vi "PacificPowerSource.vi"() -> ()   [LabVIEW 2018, in "Visualization.lvlib" / "VisualizeAcPwr.lvclass"]
doc: "This VI listens for any measurement data associated with the provided PluginName and displays it to the user for analysis. The display is only suitable for data coming from the RoomAlert Plugin."
uses:
  VisualizeAcPwr.lvclass
  ChromaPowerSupply/Loop Parameters.ctl
  VisualizeBase/VisualizeBase_class/SubVIs/VisualizationOptions.ctl
  <vilib>/Utility/miscctls.llb/LVRectTypeDef.ctl
  AcPwr/AcPwrPlugins/PacificPowerSourceClass/TypeDefs/Device(s)Settings.ctl
  AcPwr/AcPwrPlugins/PacificPowerSourceClass/TypeDefs/Measurements.ctl
  AcPwr/AcPwrPlugins/PacificPowerSourceClass/TypeDefs/MeasurementType.ctl
  AcPwr/AcPwrShared/clMeasurmentData.ctl
  AcPwr/AcPwrPlugins/AcPwrBaseClass/TypeDefs/SetParameterInputs.ctl
  <vilib>/event_ctls.llb/usereventprio.ctl
  VisualizeBase/VisualizeBase_class/Requests/VisUserEventType.ctl
  <vilib>/Utility/error.llb/Error Cluster From Error Code.vi
  <vilib>/ErrorRing/Error Ring.xnode
  <userlib>/NIST/NISTErrorLib/NISTErrorLib.lvlib
  VisualizeBase/VisualizeBase_class/VisualizeBase.lvclass
  TestClass/Test.lvclass
  Sensor/VisualizeSensor.lvclass
  StatusAndLog/VisualizeStatus.lvclass
  AcPwr/AcPwrShared/AcPwrShared.lvlib
  AcPwr/AcPwrModule/AcPwrModule.lvlib
  AcPwr/AcPwrPlugins/AcPwrPlugins.lvlib
  AcPwr/AcPwrPlugins/AcPwrBaseClass/AcPwrBase.lvclass
  AcPwr/AcPwrPlugins/PacificPowerSourceClass/PacificPowerSource.lvclass
panel:
  out "Chart#":i32
  out "MeasChannels":string[](array[string])
  out "Writetime":u32 caption="Sample Write Time(ms)"
  out "ExitHelperLoops?":bool
  in  "Display":enum16{"Raw Data", "Voltage Vs Current"}(ring)
  in  "btnPause":bool
  in  "INIFilePath":path
  in  "ModuleID":i32
  in  "Log Data":bool=TRUE
  in  "btnStop":bool
  in  "btnReset":bool
  in  "btnClearTest":bool
  in  "btnStopModule":bool
  out "XY Graph":cluster{dbl[], dbl[]}(graph)
  out "Chart":waveform(dbl)[](graph)=[{"t0"=timestamp(3657200531.6397257 s since 1904-01-01), "dt"=1.0, "Y"=[46.19]}, {"t0"=timestamp(3657200531.6397257 s since 1904-01-01), "dt"=1.0, "Y"=[2.0]}, {"t0"=timestamp(3657200531.6397257 s since 1904-01-01), "dt"=1.0, "Y"=[60.0]}]
  in  "Current":bool
  in  "Voltage":bool
  in  "Current (A)":dbl
  in  "Voltage (V)":dbl
  in  "btnStopParameterLoop":bool
  in  "btnRunParamLoop":bool
  in  "Loop Parameters":T1={"Parameter"=enum."Voltage", "Start Value"=5.0, "Increment"=1.0, "Interval (s)"=3.0, "# Iterations"=6, "End Value"=10.0} {"# Iterations" min=1; "Increment" format="%#.4f"}
  out "ErrorArray":errorcluster[](array[cluster])
  out "Incorrect DataType?":bool
  out "String Results":string
  in  "PluginName":string="Sensor.RoomAlert1"
  # "Set Parameter"
  # "Parameter Looping"
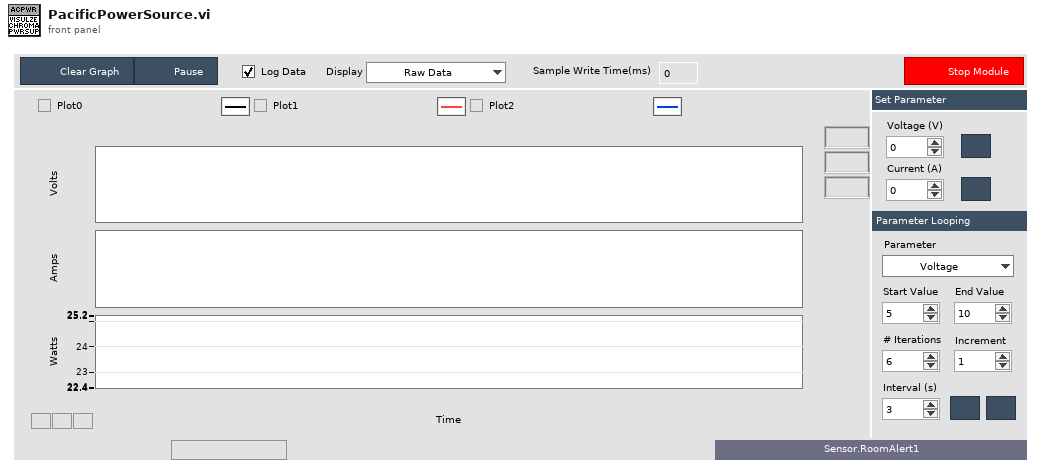
[diagram p1: front panel]
types:
  T1 = typedef "Loop Parameters.ctl" = cluster{"Parameter":enum16{"Voltage", "Current", "Power", "Resistance"}, "Start Value":dbl, "Increment":dbl, "Interval (s)":dbl, "# Iterations":u32, "End Value":dbl}
  T2 = typedef "Visualization.lvlib/VisualizeBase.lvclass/VisualizationOptions.ctl" = cluster{"PauseAtStartup":bool, "LogData":bool, "LaunchInSubPanel":bool, "FPMonitor":u16, "FPWindowBounds":T3, "MonitorBounds":cluster{"Left":i16, "Top":i16, "Right":i16, "Bottom":i16}, "MeasIndices":i32[]}
  T3 = typedef "LVRectTypeDef.ctl" = cluster{"Left":i16, "Top":i16, "Right":i16, "Bottom":i16}
  T4 = enum16{"open", "open or create", "create or replace", "create", "open (read-only)"}
  T5 = typedef "Visualization.lvlib/VisualizeBase.lvclass/VisRequestEvents.ctl" = cluster{"StopRequest":refnum<user-event>, "ResetRequest":refnum<user-event>, "FP Pop In or Out":refnum<user-event>}
  T6 = typedef "AcPwrShared.lvlib/AcPwrBroadcastEvents.ctl" = cluster{"DidInit":refnum<user-event>, "StatusUpdate":refnum<user-event>, "ErrorReport":refnum<user-event>, "DidStop":refnum<user-event>, "PathToINI":refnum<user-event>, "Measurements":refnum<user-event>, "LoadConfigFile":refnum<user-event>, "GetSettings":refnum<user-event>, "SetSettings":refnum<user-event>, "GetType&ID":refnum<user-event>, "GotSettings":refnum<user-event>, "GotSettingsLV":refnum<user-event>, "ParameterSet":refnum<user-event>}
  T7 = typedef "Visualization.lvlib/VisualizeBase.lvclass/VisFrmWrkBroadcastEvents.ctl" = cluster{"StatusUpdate":refnum<user-event>, "DidStop":refnum<user-event>, "NewModuleLoaded":refnum<user-event>, "StopVisualization":refnum<user-event>}
  T8 = typedef "AcPwrPlugins.lvlib/PacificPowerSource.lvclass/Device(s)Settings.ctl" = cluster{"MeasName":string, "Modules":cluster{"Handle":string, "Connected":bool, "Clear Device (F)":bool, "btnIdQuery":bool, "btnReset":bool, "Program #":cluster{"Phase B (Degrees)":i32, "Waveform A (1: Sine)":i32, "Voltage Level (Va)":dbl, "Program Number (0)":i32, "Voltage Level (Vb) ":dbl, "Form (3: Three)":u16, "Coupling  (0: Direct)":u16, "Frequency (45Hz)":dbl, "Current Limit (40A)":dbl, "Phase C (Degrees)":i32, "Voltage Level (Vc)":dbl, "Waveform B (1: Sine)":i32, "Waveform C (1: Sine)":i32}[], "Impedance Parameters (off, 0.00)":cluster{"State":bool, "Impedance":dbl}, "Transient Execution (F)":bool, "OutputEnabled":bool, "Source Range":cluster{"Frequency Minimum (45 Hz)":dbl, "Frequency Maximum (1200 Hz)":dbl, "Voltage Maximum (V)":dbl, "Voltage Minimum (V)":dbl, "Range Control (0: Auto)":u16, "Initial Voltage (0V)":dbl, "Frequency Range (600Hz)":u16}, "Port Type":enum16{"GPIB", "Serial"}}[]}
  T9 = typedef "AcPwrPlugins.lvlib/PacificPowerSource.lvclass/Measurements.ctl" = cluster{"Handle":string, "Name":string, "Enabled ":bool, "Measurement Value":dbl, "Channel Name":enum16{"A", "B", "C"}, "Measurement Type ":T10}[]
  T10 = typedef "AcPwrPlugins.lvlib/PacificPowerSource.lvclass/MeasurementType.ctl" = enum16{"Voltage RMS L-N", "Voltage RMS L-L", "Frequency", "Current RMS", "Current Peak", "Crest Factor", "Power Factor", "Power VA", "Real Power"}
  T11 = cluster{"Device(s)Settings":T8, "Measurements":T9}
  T12 = typedef "AcPwrShared.lvlib/clMeasurmentData.ctl" = cluster{"MeasName":string, "XML Data":string, "WaveformData":waveform(dbl)[]}
  T13 = typedef "AcPwrPlugins.lvlib/AcPwrBase.lvclass/SetParameterInputs.ctl" = cluster{"Type":string, "Parameter":string, "Phase":i32, "Value":dbl, "Command":string, "Time Stamp":timestamp}
  T14 = typedef "Visualization.lvlib/VisualizeBase.lvclass/VisUserEventType.ctl" = cluster{"BusIndex":i8, "Data":variant}
  T15 = typedef "usereventprio.ctl" = enum32{"high priority", "normal priority"}
  T16 = cluster{"Handle":string, "Connected":bool, "Clear Device (F)":bool, "btnIdQuery":bool, "btnReset":bool, "Program #":cluster{"Phase B (Degrees)":i32, "Waveform A (1: Sine)":i32, "Voltage Level (Va)":dbl, "Program Number (0)":i32, "Voltage Level (Vb) ":dbl, "Form (3: Three)":u16, "Coupling  (0: Direct)":u16, "Frequency (45Hz)":dbl, "Current Limit (40A)":dbl, "Phase C (Degrees)":i32, "Voltage Level (Vc)":dbl, "Waveform B (1: Sine)":i32, "Waveform C (1: Sine)":i32}[], "Impedance Parameters (off, 0.00)":cluster{"State":bool, "Impedance":dbl}, "Transient Execution (F)":bool, "OutputEnabled":bool, "Source Range":cluster{"Frequency Minimum (45 Hz)":dbl, "Frequency Maximum (1200 Hz)":dbl, "Voltage Maximum (V)":dbl, "Voltage Minimum (V)":dbl, "Range Control (0: Auto)":u16, "Initial Voltage (0V)":dbl, "Frequency Range (600Hz)":u16}, "Port Type":enum16{"GPIB", "Serial"}}[]
  T17 = cluster{"Handle":string, "Connected":bool, "Clear Device (F)":bool, "btnIdQuery":bool, "btnReset":bool, "Program #":cluster{"Phase B (Degrees)":i32, "Waveform A (1: Sine)":i32, "Voltage Level (Va)":dbl, "Program Number (0)":i32, "Voltage Level (Vb) ":dbl, "Form (3: Three)":u16, "Coupling  (0: Direct)":u16, "Frequency (45Hz)":dbl, "Current Limit (40A)":dbl, "Phase C (Degrees)":i32, "Voltage Level (Vc)":dbl, "Waveform B (1: Sine)":i32, "Waveform C (1: Sine)":i32}[], "Impedance Parameters (off, 0.00)":cluster{"State":bool, "Impedance":dbl}, "Transient Execution (F)":bool, "OutputEnabled":bool, "Source Range":cluster{"Frequency Minimum (45 Hz)":dbl, "Frequency Maximum (1200 Hz)":dbl, "Voltage Maximum (V)":dbl, "Voltage Minimum (V)":dbl, "Range Control (0: Auto)":u16, "Initial Voltage (0V)":dbl, "Frequency Range (600Hz)":u16}, "Port Type":enum16{"GPIB", "Serial"}}
  T18 = cluster{"Phase B (Degrees)":i32, "Waveform A (1: Sine)":i32, "Voltage Level (Va)":dbl, "Program Number (0)":i32, "Voltage Level (Vb) ":dbl, "Form (3: Three)":u16, "Coupling  (0: Direct)":u16, "Frequency (45Hz)":dbl, "Current Limit (40A)":dbl, "Phase C (Degrees)":i32, "Voltage Level (Vc)":dbl, "Waveform B (1: Sine)":i32, "Waveform C (1: Sine)":i32}[]
  T19 = cluster{"Phase B (Degrees)":i32, "Waveform A (1: Sine)":i32, "Voltage Level (Va)":dbl, "Program Number (0)":i32, "Voltage Level (Vb) ":dbl, "Form (3: Three)":u16, "Coupling  (0: Direct)":u16, "Frequency (45Hz)":dbl, "Current Limit (40A)":dbl, "Phase C (Degrees)":i32, "Voltage Level (Vc)":dbl, "Waveform B (1: Sine)":i32, "Waveform C (1: Sine)":i32}
  T20 = typedef "sizeaction.ctl" = enum32{"Minimized", "Maximized", "Resized"}
  T21 = typedef "LVPoint32TypeDef.ctl" = cluster{"Horizontal":i32, "Vertical":i32}
  T22 = enum16{"Voltage", "Current", "Power", "Resistance"}
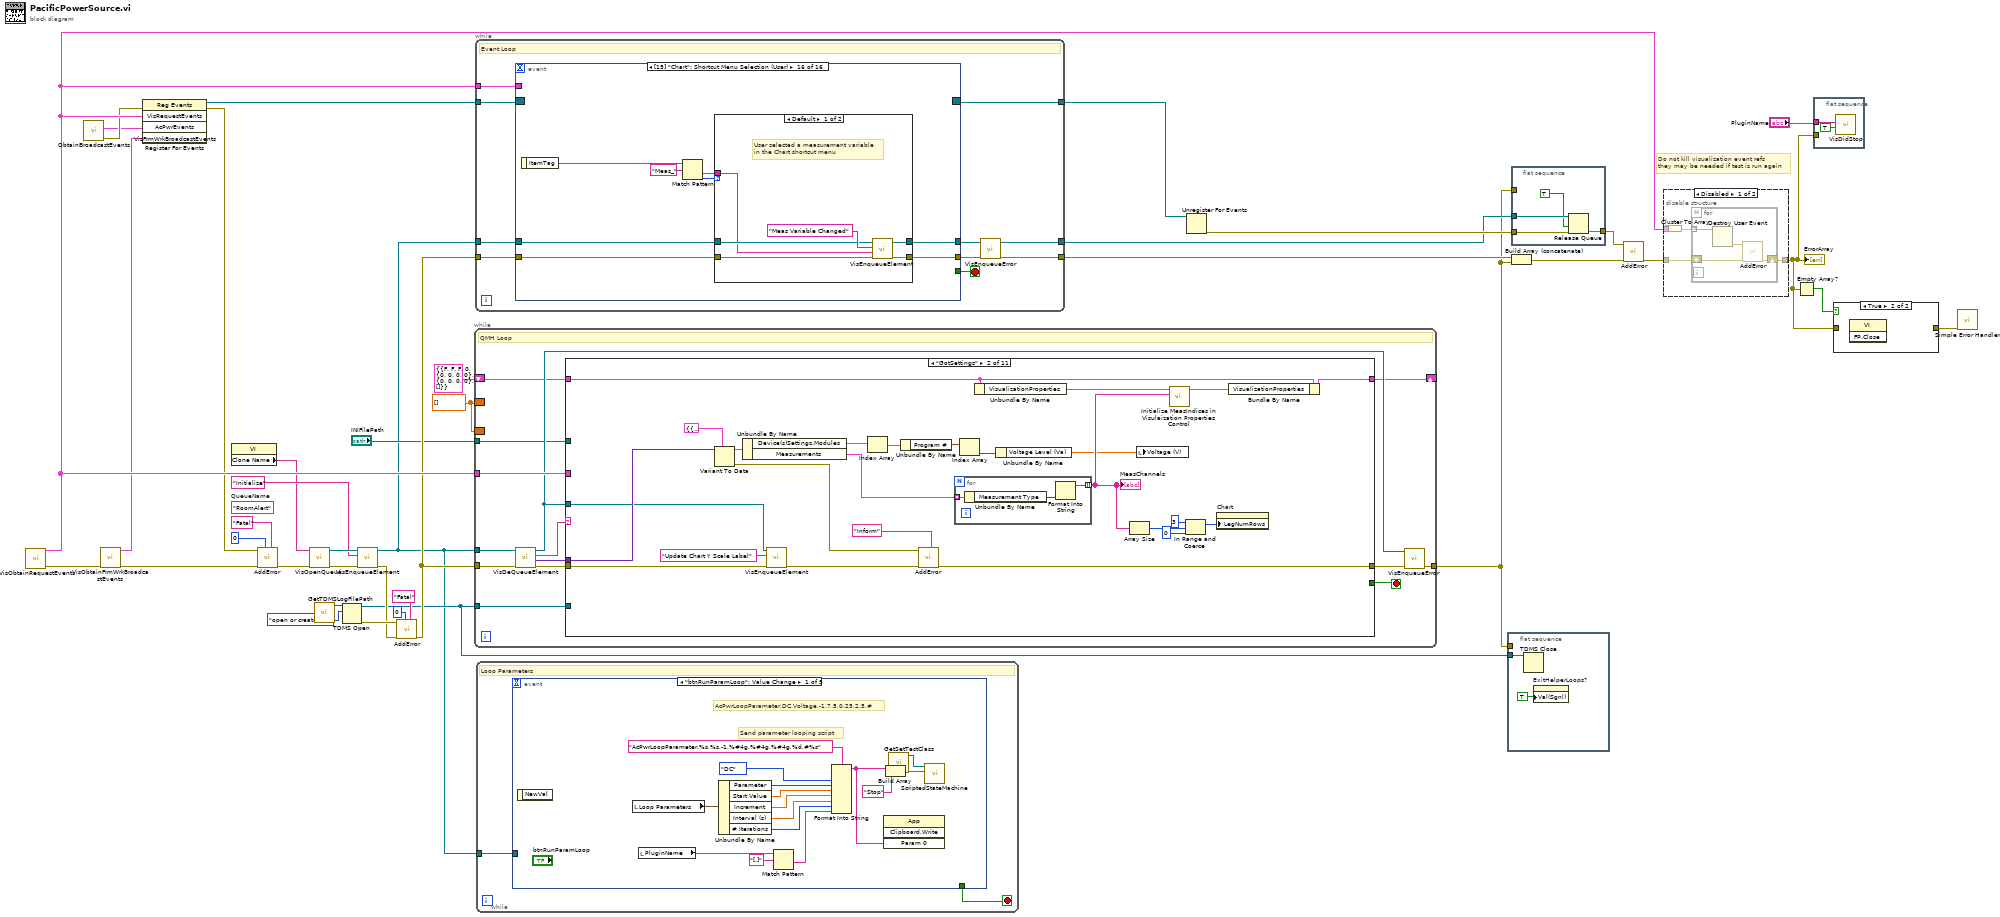
[diagram p0: block diagram]
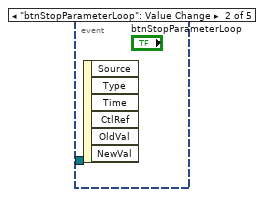
[diagram p2: hidden frame]
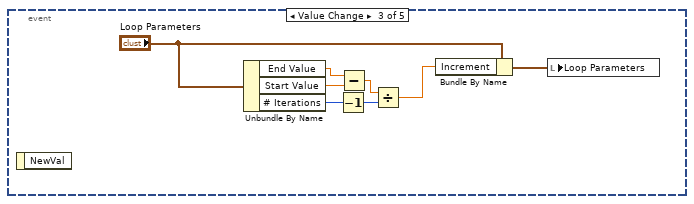
[diagram p3: hidden frame]
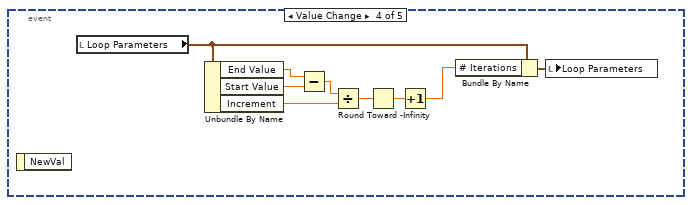
[diagram p4: hidden frame]
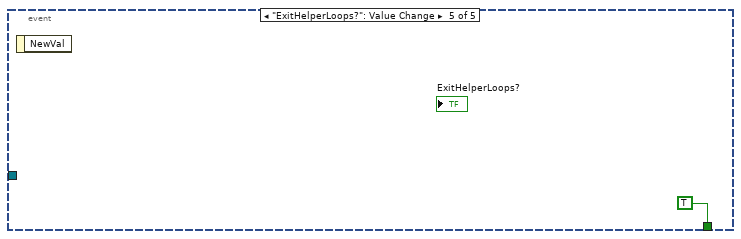
[diagram p5: hidden frame]
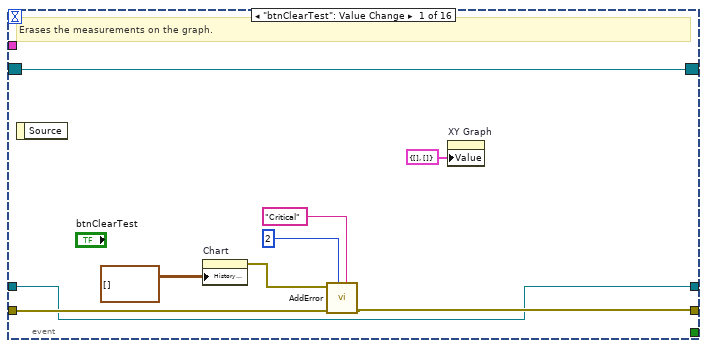
[diagram p7: hidden frame]
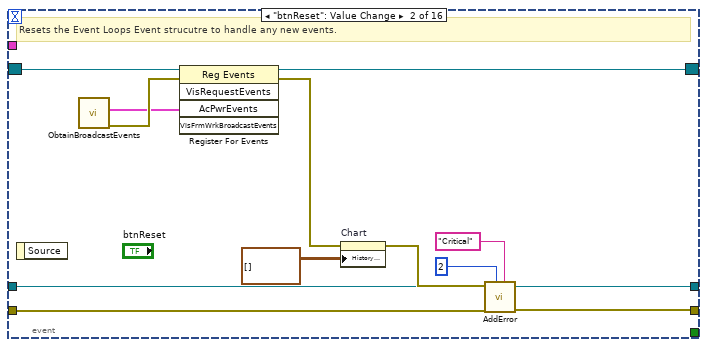
[diagram p8: hidden frame]
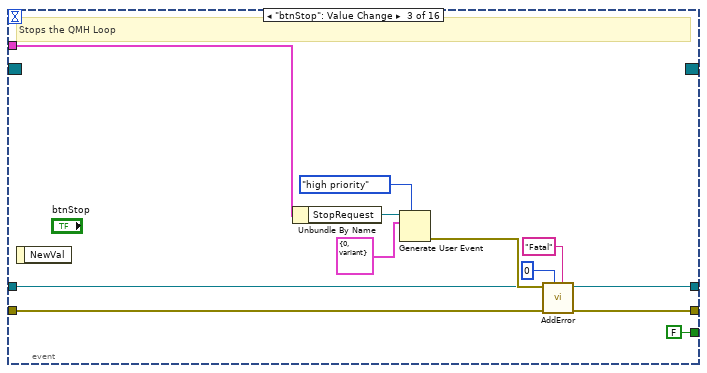
[diagram p9: hidden frame]
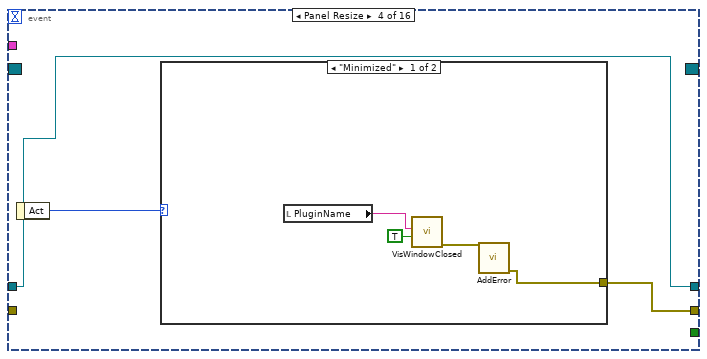
[diagram p10: hidden frame]
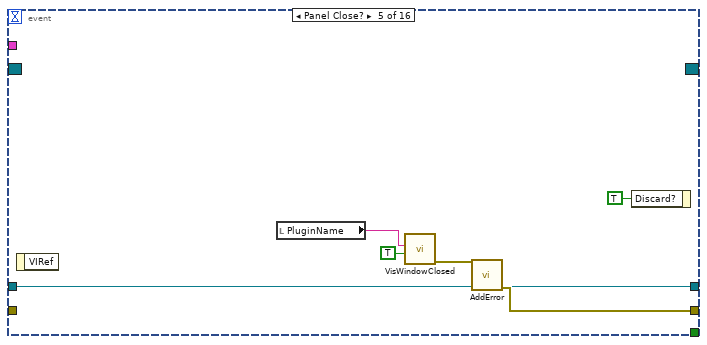
[diagram p12: hidden frame]
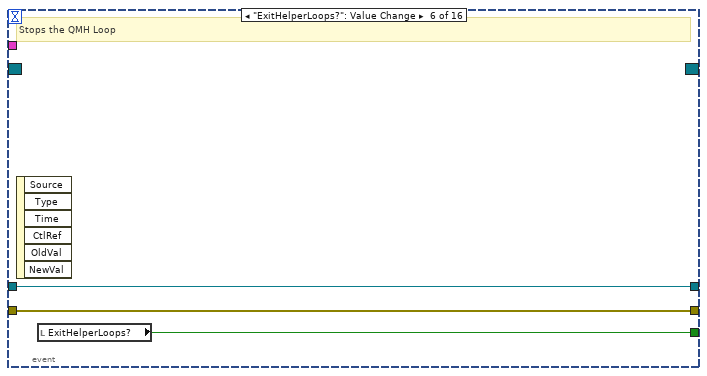
[diagram p13: hidden frame]
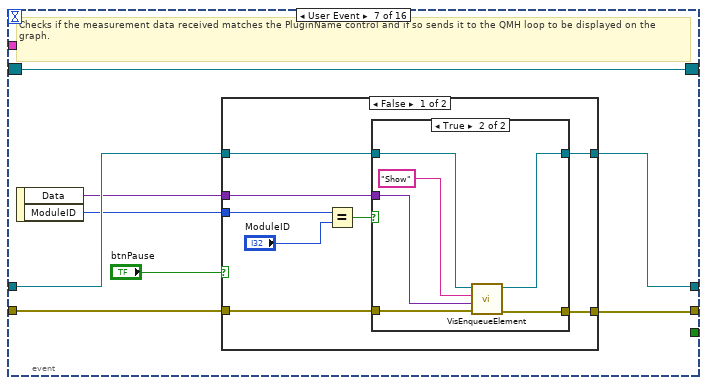
[diagram p14: hidden frame]
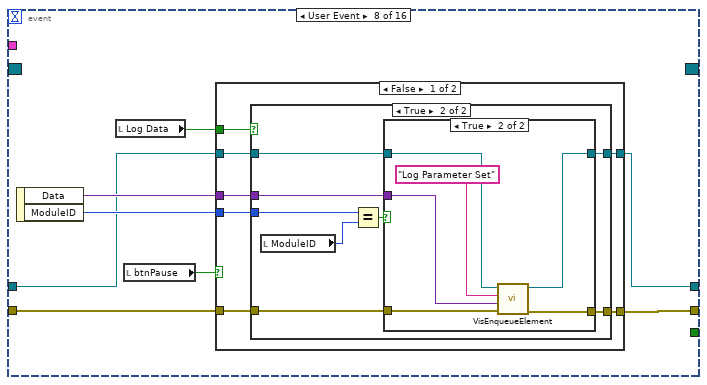
[diagram p17: hidden frame]
diagram:
  w2 = dbl[] []
  (unwired) "RoomAlert"  # QueueName
  # "Do not kill visualization event refs\nthey may be needed if test is run again"
  n1 = call "VisObtainRequestEvents.vi"() -> ("Error"=w30:errorcluster[], "VisRequestEvents"=w32:T5)  [unwired: 10 in]
  n2 = call "ObtainBroadcastEvents.vi"() -> ("error out"=w26:errorcluster, "AcPwrEvents"=w19:T6)  [unwired: 10 in]
  n3 = call "VisObtainFrmWrkBroadcastEvents.vi"("Error"=w30) -> ("Error"=w5:errorcluster[], "VisFrmWrkBroadcastEvents"=w4:T7)  [unwired: 9 in]
  n4 = register-events(error in=w26, w32, w19, w4) -> (reference out=w39:refnum<event-registration>, error out=w29:errorcluster)  [unwired: 1 in]
  n5 = property class="VI"() -> ("Clone Name"=w18:string)  [unwired: 2 in, 2 out]
  n6 = call <userlib>:"AddError.vi"("Severity"="Fatal", "Priority"=u8 0, "ErrorArray In"=w5, "error in (no error)"=w29) -> ("ErrorArray Out"=w25:errorcluster[])  [unwired: 6 in, 1 out]
  n7 = call "VisOpenQueue.vi"("Error Array In"=w25, "QueueName"=w18) -> ("Error Array Out"=w23:errorcluster[], "queue out"=w24:refnum<queue>)  [unwired: 8 in]
  n8 = call "GetTDMSLogFilePath.vi"() -> ("TDMS Log File Path"=w17:path)  [unwired: 11 in]
  n9 = TDMS Open(10:T4."open or create" ("operation (0:open)"), 11:w17) -> (0:w14:errorcluster, 3:w10:refnum<k34>)  [unwired: 5 in]
  n10 = call "VisEnqueueElement.vi"("Error Array In"=w23, "Message"="Initialize", "queue in"=w24) -> ("Error Array Out"=w13:errorcluster[], "queue out"=w3:refnum<queue>)  [unwired: 7 in]
  n11 = call <userlib>:"AddError.vi"("Severity"="Fatal", "Priority"=u8 0, "ErrorArray In"=w13, "error in (no error)"=w14) -> ("ErrorArray Out"=w12:errorcluster[])  [unwired: 6 in, 1 out]
  n12 = while {
    tunnel: w12 -> [w47]
    tunnel: [w50] -> w9
    tunnel: w3 -> [w46]
    tunnel: w32 -> [w52]
    tunnel: w10 -> [w43]
    tunnel: "INIFilePath" -> [w42]
    border: w2 -> [_]
    border: w2 -> [_]
    shift-right: [w40] -> _
    shift-left: cluster{"VisualizationProperties":T2} {"VisualizationProperties"={"PauseAtStartup"=FALSE, "LogData"=FALSE, "LaunchInSubPanel"=FALSE, "FPMonitor"=0, "FPWindowBounds"={"Left"=0, "Top"=0, "Right"=0, "Bottom"=0}, "MonitorBounds"={"Left"=0, "Top"=0, "Right"=0, "Bottom"=0}, "MeasIndices"=[]}} ("output cluster") -> [w41]
    stop <- w53 stop-if-true
    # "QMH Loop"
    n13 = call "VisDeQueueElement.vi"("Error Array In"=w47, "Queue In"=w46) -> ("Error Array Out"=w45:errorcluster[], "Data"=w48:variant, "Message"=w49:string, "Queue Out"=w44:refnum<queue>)  [unwired: 6 in]
    n14 = case shown="\"GotSettings\"" w49 {
      selector: w49 -> [_ _ _ _ _ _ w227 _ _ _ _]
      tunnel: w48 -> [_ w91 _ w112 w128 w202 _ w247 _ _ w292]
      tunnel: w45 -> [w66 w74 _ w109 w129 _ w225 _ w277 _ w287]
      tunnel: [w60 w90 _ w108 w130 _ w224 w237 w276 _ w289] -> w51
      tunnel: [_ _ _ _ _ _ _ w243 TRUE _ _] -> w53
      tunnel: w52 -> [_ _ _ _ _ _ _ w242 _ _ _]
      tunnel: w44 -> [_ w76 _ w110 _ _ _ w241 _ _ _]
      tunnel: w43 -> [_ _ _ _ w127 w201 _ _ _ _ _]
      tunnel: w42 -> [w65 _ _ _ _ _ _ _ w278 _ _]
      tunnel: w41 -> [w56 w82 w99 w119 w120 w199 w220 w235 w275 w282 w283]
      tunnel: [w55 w81 w99 w118 w120 w199 w220 w235 w275 w282 w283] -> w40
      frame "Initialize" {
        n15 = property on="Chart" class="WFChart (strict)"("History Data"=waveform(dbl)[][] []) -> ()  [unwired: 2 in, 2 out]
        n16 = property on="XY Graph" class="XYGraph (strict)"("Value"=cluster{dbl[], dbl[]} {[], []} ("XY Graph")) -> ()  [unwired: 2 in, 2 out]
        n17 = call "ApplyVisOptions.vi"("INIFilePath"=w65) -> ("error out"=w69:errorcluster, "VisualizationProperties"=w54:T2)  [unwired: 9 in]
        n18 = Bundle By Name(cluster=w56, "VisualizationProperties"=w54) -> (w55:cluster{"VisualizationProperties":T2})
        n19 = call <userlib>:"AddError.vi"("Severity"="Inform", "ErrorArray In"=w66, "error in (no error)"=w69) -> ("ErrorArray Out"=w67:errorcluster[])  [unwired: 7 in, 1 out]
        n20 = property on="Display" class="Enum (strict)"("Val(Sgnl)"="Display") -> ()  [unwired: 2 in, 2 out]
        n21 = local read "ModuleID"() -> (w57:i32)
        n22 = call "GetSettingsRequestLV.vi"("SettingsToGet"=variant, "ModuleID"=w57) -> ("Error Out"=w59:errorcluster)  [unwired: 9 in]
        n23 = call <userlib>:"AddError.vi"("Severity"="Inform", "ErrorArray In"=w67, "error in (no error)"=w59) -> ("ErrorArray Out"=w60:errorcluster[])  [unwired: 7 in, 1 out]
      }
      frame "GotSettings" {
        n24 = Variant To Data(type=T11 {"Device(s)Settings"={"MeasName"="", "Modules"=[]}, "Measurements"=[]} ("output cluster"), Variant=w91) -> (data=w92:T11, error out=w89:errorcluster)  [unwired: 1 in]
        n25 = Unbundle By Name(w92) -> ("Device(s)Settings.Modules"=w93:T16, "Measurements"=w84:T9)
        n26 = call "VisEnqueueElement.vi"("Error Array In"=w74, "Message"="Update Chart Y Scale Label", "queue in"=w76) -> ("Error Array Out"=w75:errorcluster[])  [unwired: 7 in, 1 out]
        n27 = Index Array(array=w93) -> (element=w94:T17)  [unwired: 1 in]
        n28 = Unbundle By Name(w94) -> ("Program #"=w72:T18)
        n29 = call <userlib>:"AddError.vi"("Severity"="Inform", "ErrorArray In"=w75, "error in (no error)"=w89) -> ("ErrorArray Out"=w90:errorcluster[])  [unwired: 7 in, 1 out]
        n30 = for {
          tunnel: w84 -> [w97] mode=indexing
          tunnel: [w95] -> w78 mode=indexing
          n31 = Unbundle By Name(w97) -> ("Measurement Type"=w96:T10)
          n32 = Format Into String(w96) -> (resulting string=w95:string)  [unwired: 3 in, 1 out]
        }
        "MeasChannels" <- w78
        n33 = Index Array(array=w72) -> (element=w71:T19)  [unwired: 1 in]
        n34 = Unbundle By Name(w82) -> ("VisualizationProperties"=w79:T2)
        n35 = Unbundle By Name(w71) -> ("Voltage Level (Va)"=w70:dbl)
        n36 = Array Size(array=w78) -> (size(s)=w87:i32)
        n37 = local write "Voltage (V)"(w70) -> ()
        n38 = call "Initialize MeasIndices in Visulaization Properties Control.vi"("MeasChannels"=w78, "VisualizationProperties"=w79) -> ("VisualizationProperties out"=w80:T2)  [unwired: 8 in, 1 out]
        n39 = In Range and Coerce(upper limit=3, x=w87, lower limit=0) -> (coerced(x)=w83:i32)  [unwired: 1 out]
        n40 = property on="Chart" class="WFChart (strict)"("LegNumRows"=w83) -> ()  [unwired: 2 in, 2 out]
        n41 = Bundle By Name(cluster=w82, "VisualizationProperties"=w80) -> (w81:cluster{"VisualizationProperties":T2})
      }
      frame "Update Chart Y Scale Label" {
        n42 = Unbundle By Name(w99) -> ("VisualizationProperties.MeasIndices"=w100:i32[])
        n43 = control-ref of="Chart"() -> (w102:refnum<vi>)
        n44 = local read "MeasChannels"() -> (w101:string[])
        n45 = for {
          tunnel: w100 -> [w105] mode=indexing
          tunnel: w102 -> [w107]
          tunnel: w101 -> [w106]
          i -> [w104]
          n46 = Index Array(array=w106, index=w105) -> (element=w103:string)
          n47 = property class="WFChart (strict)"(reference=w107, "ActYScl"=w104, "YScale.NameLbl.Text"=w103, "Active Plot"=w104, "Plot.Plot Name"=w103) -> ()  [unwired: 1 in, 2 out]
        }
        n48 = property on="Chart" class="WFChart (strict)"("History Data"=waveform(dbl)[][] []) -> ()  [unwired: 2 in, 2 out]
      }
      frame "Meas Variable Changed" {
        n49 = Unbundle By Name(w119) -> ("VisualizationProperties"=w117:T2)
        n50 = Variant To Data(type="" ("Message"), Variant=w112) -> (data=w111:string)  [unwired: 1 in, 1 out]
        n51 = local read "Chart#"() -> (w115:i32)
        n52 = call "Update MeasIndices in Visualization Properties Control.vi"("Item Tag"=w111, "Chart# user clicked on"=w115, "VisualizationProperties In"=w117) -> ("VisualizationProperties"=w116:T2)  [unwired: 8 in]
        n53 = Bundle By Name(cluster=w119, "VisualizationProperties"=w116) -> (w118:cluster{"VisualizationProperties":T2})
        n54 = call "VisEnqueueElement.vi"("Error Array In"=w109, "Message"="Update Chart Y Scale Label", "queue in"=w110) -> ("Error Array Out"=w108:errorcluster[])  [unwired: 7 in, 1 out]
      }
      frame "Show" {
        n55 = flat-sequence {
          tunnel: w127 -> [w132]
          tunnel: w128 -> [w133]
          tunnel: w129 -> [w134]
          tunnel: [w134] -> w126
          tunnel: [w133] -> w125
          tunnel: [w132] -> w124
          tunnel: [w131] -> w123
          tunnel: w126 -> [w150]
          tunnel: w125 -> [w149]
          tunnel: w124 -> [w144]
          tunnel: w123 -> [w137]
          tunnel: [w151] -> w122
          tunnel: [w137] -> w121
          tunnel: w120 -> [w136]
          tunnel: [w198] -> w130
          tunnel: w122 -> [w198]
          tunnel: w121 -> [w196]
          frame #0 {
            n56 = Tick Count (ms)() -> (millisecond timer value=w131:u32)
          }
          frame #1 {
            w146 = u32[] [0, 1, 2]  # PlotYAxis
            n57 = Variant To Data(type=T12 {"MeasName"="", "XML Data"="", "WaveformData"=[]} ("MeasurmentDataCluster"), Variant=w149) -> (data=w147:T12, error out=w148:errorcluster)  [unwired: 1 in]
            n58 = Unbundle By Name(w136) -> ("VisualizationProperties.MeasIndices"=w135:i32[])
            n59 = control-ref of="Chart"() -> (w138:refnum<vi>)
            n60 = Unbundle By Name(w147) -> ("WaveformData"=w139:waveform(dbl)[])
            n61 = call "RetrieveAcPwrMeasurementData.vi"("WaveformChartReference"=w138, "PlotYScale"=w146, "WaveformArrayIn"=w139, "error in (no error)"=w148) -> ("WaveformArrayOut"=w141:waveform(dbl)[], "OutputString(Chroma)"=w143:string, "Incorrect DataType?"=w142:bool, "error out"=w145:errorcluster)  [unwired: 7 in, 1 out]
            n62 = case shown="False" w142 {
              selector: w142 -> [w166 _]
              tunnel: [w175 w194] -> w151
              tunnel: w150 -> [w174 w194]
              tunnel: w145 -> [w171 _]
              tunnel: w144 -> [w168 _]
              tunnel: w143 -> [w167 _]
              tunnel: w141 -> [w154 _]
              tunnel: w135 -> [w152 _]
              frame False {
                n63 = for {
                  tunnel: w154 -> [w178]
                  tunnel: w152 -> [w177] mode=indexing
                  tunnel: [w176] -> w153 mode=indexing
                  n64 = Index Array(array=w178, index=w177) -> (element=w176:waveform(dbl))
                }
                "Chart" <- w153
                n65 = Index Array(array=w154, index #1=1 ("index"), index #2=0 ("index")) -> (element #1=w165:waveform(dbl), element #2=w164:waveform(dbl))
                n66 = Unbundle By Name(w165) -> ("Y"=w163:dbl[])
                n67 = Unbundle By Name(w164) -> ("Y"=w160:dbl[])
                n68 = feedback #1() -> (w162:dbl[])
                n69 = Build Array (concatenate)(w162, w163) -> (w157:dbl[])
                n70 = feedback-in #1(w157) -> ()
                n71 = feedback #2() -> (w161:dbl[])
                n72 = Build Array (concatenate)(w161, w160) -> (w156:dbl[])
                n73 = feedback-in #2(w156) -> ()
                n74 = Bundle(w157, w156) -> (→"XY Graph":cluster{dbl[], dbl[]})  [unwired: 1 in]
                n75 = case shown="True" "Log Data" {
                  tunnel: w171 -> [w179 w192]
                  tunnel: [w179 w193] -> w170
                  tunnel: w154 -> [_ w191]
                  tunnel: w168 -> [_ w186]
                  frame False {
                  }
                  frame True {
                    n76 = call "PrepareWaveformDataForTDMS.vi"("error in (no error)"=w192, "WaveformArray in"=w191) -> ("error out"=w190:errorcluster, "Measurement Data"=w188:dbl[][], "Channel Names"=w189:string[], "TimeStamp"=w181:timestamp)  [unwired: 6 in]
                    n77 = local read "PluginName"() -> (w184:string)
                    n78 = Build Array(w181) -> (w180:timestamp[])
                    n79 = TDMS Write(0:w186, 5:w184, 7:"TimeStamp" ("PluginName"), 9:w180, 11:w190) -> (4:w185:refnum<k34>, 6:w183:string, 15:w187:errorcluster)  [unwired: 1 in, 1 out]
                    n80 = TDMS Write(0:w185, 5:w183, 7:w189, 9:w188, 11:w187) -> (15:w193:errorcluster)  [unwired: 1 in, 3 out]
                  }
                }
                n81 = call <userlib>:"AddError.vi"("Severity"="Fatal" ("String"), "Priority"=u8 0, "ErrorArray In"=w174, "error in (no error)"=w170) -> ("ErrorArray Out"=w175:errorcluster[])  [unwired: 6 in, 1 out]
                "String Results" <- w167
                "Incorrect DataType?" <- w166
              }
              frame True {
              }
            }
          }
          frame #2 {
            n82 = Tick Count (ms)() -> (millisecond timer value=w197:u32)
            n83 = Subtract(x=w197, y=w196) -> (x-y=→"Writetime":u32)
          }
        }
      }
      frame "Log Parameter Set" {
        n84 = Variant To Data(type=T13 {"Type"="", "Parameter"="", "Phase"=0, "Value"=0.0, "Command"="", "Time Stamp"=timestamp(0 s since 1904-01-01)}, Variant=w202) -> (data=w214:T13, error out=w203:errorcluster)  [unwired: 1 in]
        n85 = Unbundle By Name(w214) -> ("Type"=w213:string, "Parameter"=w212:string, "Phase"=w211:i32, "Time Stamp"=w207:timestamp, "Value"=w205:dbl)
        n86 = local read "PluginName"() -> (w200:string)
        n87 = Format Into String(format string="Set-%s_%s_Phase_%d", w213, w212, w211) -> (resulting string=w206:string)  [unwired: 2 in, 1 out]
        n88 = Concatenate Strings(w206, "_TimeStamp" ("string")) -> (w208:string)
        n89 = Build Array(w207) -> (w215:timestamp[])
        n90 = Build Array(w205) -> (w204:dbl[])
        n91 = TDMS Write(0:w201, 5:w200, 7:w208, 9:w215, 11:w203) -> (4:w217:refnum<k34>, 6:w216:string, 15:w218:errorcluster)  [unwired: 1 in, 1 out]
        n92 = TDMS Write(0:w217, 5:w216, 7:w206, 9:w204, 11:w218) -> ()  [unwired: 1 in, 4 out]
      }
      frame Default {
        n93 = xnode "Error Ring"("parameter 0"=w227) -> ("error out"=w226:errorcluster)
        n94 = call <userlib>:"AddError.vi"("Severity"="Inform" ("String"), "Priority"=u8 5, "ErrorArray In"=w225, "error in (no error)"=w226) -> ("ErrorArray Out"=w224:errorcluster[], "error out"=w223:errorcluster)  [unwired: 6 in]
        n95 = call <vilib>:"Clear Errors.vi"("error in (no error)"=w223) -> ()  [unwired: 5 in, 2 out]
      }
      frame "Error" {
        n96 = Variant To Data(type=errorcluster[] [], Variant=w247) -> (data=w245:errorcluster[], error out=w236:errorcluster)  [unwired: 1 in]
        n97 = call <userlib>:"ParseErrors.vi"("ErrorArray"=w245) -> ("ErrorArray"=w244:errorcluster[])  [unwired: 8 in, 2 out]
        n98 = for {
          tunnel: w244 -> [w258] mode=indexing
          tunnel: [w252] -> w238 mode=concatenating
          tunnel: [w250] -> w243
          tunnel: w242 -> [w249]
          tunnel: w241 -> [w248]
          stop <- w250 stop-if-true
          n99 = call <userlib>:"GeneralHandler.vi"("error in (no error)"=w258) -> ("Severity"=w251:string, "Stop"=w255:bool, "Abort"=w256:bool, "Continue"=w257:bool)  [unwired: 6 in, 1 out]
          n100 = Build Array(w257, w256, w255) -> (w254:bool[])
          n101 = Boolean Array To Number(Boolean array=w254) -> (number=w253:u32)
          n102 = case shown="1" w253 {
            tunnel: [_ _ w263 w272] -> w252
            tunnel: w251 -> [_ _ _ w265]
            tunnel: [_ _ _ w267] -> w250
            tunnel: w249 -> [_ _ _ w266]
            tunnel: w248 -> [_ _ w259 _]
            frame 0, Default {
              # "No Dialog"
            }
            frame 1 {
              # "Continue"
            }
            frame 2 {
              # "Abort, Flush Queue"
              n103 = Flush Queue(queue=w259) -> (error out=w262:errorcluster)  [unwired: 1 in, 2 out]
              n104 = call <userlib>:"AddError.vi"("Severity"="Critical" ("String"), "Priority"=u8 1, "error in (no error)"=w262) -> ("ErrorArray Out"=w263:errorcluster[])  [unwired: 7 in, 1 out]
            }
            frame 4 {
              # "Stop"
              n105 = Unbundle By Name(w266) -> ("StopRequest"=w273:refnum<user-event>)
              n106 = Equal?(x=w265, y="Fatal" ("x")) -> (x = y?=w267:bool)
              n107 = Generate User Event(priority (normal)=usereventprio."high priority", user event=w273, event data cluster=T14 {"BusIndex"=0, "Data"=variant} ("event data")) -> (error out=w271:errorcluster)  [unwired: 1 in, 1 out]
              n108 = call <userlib>:"AddError.vi"("error in (no error)"=w271) -> ("ErrorArray Out"=w272:errorcluster[], "error out"=w268:errorcluster)  [unwired: 9 in]
              n109 = call <vilib>:"Clear Errors.vi"("error in (no error)"=w268) -> ()  [unwired: 5 in, 2 out]
            }
          }
        }
        n110 = call <userlib>:"AddError.vi"("Severity"="Critical", "Priority"=u8 2, "ErrorArray In"=w238, "error in (no error)"=w236) -> ("ErrorArray Out"=w237:errorcluster[])  [unwired: 6 in, 1 out]
      }
      frame "Stop" {
        n111 = Unbundle By Name(w275) -> ("VisualizationProperties"=w274:T2)
        n112 = call "WriteVisOptionsToINIFile.vi"("Visualization Options"=w274, "INIFilePath"=w278) -> ("error out"=w279:errorcluster)  [unwired: 8 in, 1 out]
        n113 = call <userlib>:"AddError.vi"("Severity"="Inform", "ErrorArray In"=w277, "error in (no error)"=w279) -> ("ErrorArray Out"=w276:errorcluster[])  [unwired: 7 in, 1 out]
      }
      frame "- ---AcPwr Module Specific Commands----" {
      }
      frame "Set Parameter" {
        n114 = Variant To Data(type="", Variant=w292) -> (data=w290:string, error out=w288:errorcluster)  [unwired: 1 in]
        n115 = call <userlib>:"AddError.vi"("Severity"="Inform", "Priority"=u8 0, "ErrorArray In"=w287, "error in (no error)"=w288) -> ("ErrorArray Out"=w284:errorcluster[])  [unwired: 6 in, 1 out]
        n116 = local read "PluginName"() -> (w300:string)
        n117 = case shown="\"False\", Default" w290 {
          tunnel: "Voltage (V)" -> [_ w311 _]
          tunnel: "Current (A)" -> [_ _ w312]
          tunnel: [_ w311 w312] -> w302
          tunnel: [TRUE _ _] -> w299
          frame "False", Default {
          }
          frame "Voltage" {
          }
          frame "Current" {
          }
        }
        n118 = Match Pattern(string=w300, regular expression="[.]") -> (after substring=w301:string)  [unwired: 1 in, 3 out]
        n119 = Format Into String(format string="AcPwrSetParameter,%s,%s,-1,%.4f,#%s", enum16{"AC", "DC"}."DC" ("input 1"), w290, w302, w301) -> (resulting string=w298:string)  [unwired: 2 in, 1 out]
        n120 = case shown="False" w299 {
          tunnel: w298 -> [w307 _]
          tunnel: [w305 w309] -> w289
          tunnel: w284 -> [w303 w309]
          frame False {
            n121 = call "GetSetTestClass.vi"() -> ("Test.lvclass"=w308:refnum<class "Test.lvclass">)  [unwired: 11 in]
            n122 = Build Array(w307, "Stop" ("element")) -> (w306:string[])
            n123 = call "ScriptedStateMachine.vi"("ErrorArray 2"=w303, "script"=w306, "Test.lvclass 2"=w308) -> ("ErrorArray"=w305:errorcluster[])  [unwired: 6 in, 2 out]
          }
          frame True {
          }
        }
      }
    }
    n124 = call "VisEnqueueError.vi"("Error Array In"=w51, "Queue in"=w44) -> ("Error Array Out"=w50:errorcluster[])  [unwired: 8 in, 1 out]
  }
  n125 = while {
    tunnel: w39 -> [w322]
    tunnel: [w316] -> w37
    tunnel: [w320] -> w38
    tunnel: w32 -> [w319]
    tunnel: w12 -> [w318]
    tunnel: w3 -> [w317]
    tunnel: [w313] -> w21
    stop <- w321 stop-if-true
    # "Event Loop"
    n126 = event shown="[15] \"Chart\": Shortcut Menu Selection (User)" {
      selector: w322 -> [w325 w343 _ _ _ _ w374 _ _ _ _ _ _ _ _ _]
      dyn-events: [w325 w342 _ _ _ _ w374 _ _ _ _ _ _ _ _ _] -> w320
      timeout: _ -> [_ _ _ _ _ _ _ _ _ _ _ _ _ _ _ _]
      tunnel: [_ _ FALSE ("Priority? (F)") _ _ w368 _ _ _ _ _ _ _ _ _ _] -> w321
      tunnel: [w328 w340 w347 w356 w363 w369 w376 w397 w435 _ w457 w465 w476 w486 _ w509] -> w315
      tunnel: w319 -> [_ _ w346 _ _ _ _ _ _ _ _ _ _ _ _ _]
      tunnel: w318 -> [w329 w341 w354 _ _ w369 w377 w399 w434 _ _ w463 _ w485 _ w511]
      tunnel: w317 -> [w323 w333 w344 w355 w362 w370 w378 w400 w437 w447 w455 w462 w475 w488 _ w512]
      tunnel: [w323 w333 w344 w355 w362 w370 w375 w398 w436 w447 w456 w464 w475 w487 _ w510] -> w314
      event "btnClearTest": Value Change {
        # "Erases the measurements on the graph."
        n127 = event-data() -> ()  [unwired: 1 in, 1 out]
        n128 = property on="Chart" class="WFChart (strict)"("History Data"=waveform(dbl)[][] []) -> (error out=w327:errorcluster)  [unwired: 2 in, 1 out]
        n129 = call <userlib>:"AddError.vi"("Severity"="Critical", "Priority"=u8 2, "ErrorArray In"=w329, "error in (no error)"=w327) -> ("ErrorArray Out"=w328:errorcluster[])  [unwired: 6 in, 1 out]
        n130 = property on="XY Graph" class="XYGraph (strict)"("Value"=cluster{dbl[], dbl[]} {[], []} ("XY Graph")) -> ()  [unwired: 2 in, 2 out]
      }
      event "btnReset": Value Change {
        # "Resets the Event Loops Event strucutre to handle any new events."
        n131 = event-data() -> ()  [unwired: 1 in, 1 out]
        n132 = call "ObtainBroadcastEvents.vi"() -> ("error out"=w334:errorcluster, "AcPwrEvents"=w332:T6)  [unwired: 10 in]
        n133 = register-events(reference=w343, error in=w334, w332) -> (reference out=w342:refnum<event-registration>, error out=w336:errorcluster)  [unwired: 2 in]
        n134 = property on="Chart" class="WFChart (strict)"(error in=w336, "History Data"=waveform(dbl)[][] []) -> (error out=w335:errorcluster)  [unwired: 1 in, 1 out]
        n135 = call <userlib>:"AddError.vi"("Severity"="Critical", "Priority"=u8 2, "ErrorArray In"=w341, "error in (no error)"=w335) -> ("ErrorArray Out"=w340:errorcluster[])  [unwired: 6 in, 1 out]
      }
      event "btnStop": Value Change {
        # "Stops the QMH Loop"
        n136 = event-data() -> ()  [unwired: 1 in, 1 out]
        n137 = Unbundle By Name(w346) -> ("StopRequest"=w352:refnum<user-event>)
        n138 = Generate User Event(priority (normal)=usereventprio."high priority", user event=w352, event data cluster=T14 {"BusIndex"=0, "Data"=variant} ("event data")) -> (error out=w353:errorcluster)  [unwired: 1 in, 1 out]
        n139 = call <userlib>:"AddError.vi"("Severity"="Fatal" ("String"), "Priority"=u8 0, "ErrorArray In"=w354, "error in (no error)"=w353) -> ("ErrorArray Out"=w347:errorcluster[])  [unwired: 6 in, 1 out]
      }
      event Panel Resize {
        n140 = event-data() -> ("Act"=w357:T20)  [unwired: 1 in]
        n141 = case shown="\"Minimized\"" w357 {
          tunnel: [w358 _] -> w356
          frame "Minimized" {
            n142 = local read "PluginName"() -> (w360:string)
            n143 = call "VisWindowClosed.vi"("Window Closed?"=TRUE ("Window Minimized or Clozed?"), "Module Name"=w360) -> ("error out"=w361:errorcluster)  [unwired: 9 in]
            n144 = call <userlib>:"AddError.vi"("error in (no error)"=w361) -> ("ErrorArray Out"=w358:errorcluster[])  [unwired: 9 in, 1 out]
          }
          frame "Maximized", Default {
          }
        }
      }
      event Panel Close? {
        n145 = event-data() -> ()  [unwired: 1 in, 1 out]
        n146 = local read "PluginName"() -> (w364:string)
        n147 = call "VisWindowClosed.vi"("Window Closed?"=TRUE ("Window Minimized or Clozed?"), "Module Name"=w364) -> ("error out"=w365:errorcluster)  [unwired: 9 in]
        n148 = call <userlib>:"AddError.vi"("error in (no error)"=w365) -> ("ErrorArray Out"=w363:errorcluster[])  [unwired: 9 in, 1 out]
        n149 = event-data("Discard?"=TRUE) -> ()  [unwired: 1 in, 1 out]
      }
      event "ExitHelperLoops?": Value Change {
        # "Stops the QMH Loop"
        n150 = event-data() -> ()  [unwired: 1 in, 6 out]
        n151 = local read "ExitHelperLoops?"() -> (w368:bool)
      }
      event User Event {
        # "Checks if the measurement data received matches the PluginName control and if so sends it to the QMH loop to be displayed on the graph."
        n152 = event-data() -> ("Data"=w373:variant, "ModuleID"=w372:i32)  [unwired: 1 in]
        n153 = case shown="False" "btnPause" {
          tunnel: w378 -> [w386 w396]
          tunnel: w377 -> [w385 w395]
          tunnel: [w384 w395] -> w376
          tunnel: [w383 w396] -> w375
          tunnel: w373 -> [w382 _]
          tunnel: w372 -> [w379 _]
          frame False {
            n154 = Equal?(x=w379, y="ModuleID") -> (x = y?=w381:bool)
            n155 = case shown="True" w381 {
              tunnel: [w387 w393] -> w384
              tunnel: w386 -> [w388 w392]
              tunnel: w385 -> [w387 w394]
              tunnel: [w388 w390] -> w383
              tunnel: w382 -> [_ w391]
              frame False {
              }
              frame True {
                n156 = call "VisEnqueueElement.vi"("Error Array In"=w394, "Data"=w391, "Message"="Show", "queue in"=w392) -> ("Error Array Out"=w393:errorcluster[], "queue out"=w390:refnum<queue>)  [unwired: 6 in]
              }
            }
          }
          frame True {
          }
        }
      }
      event User Event {
        n157 = event-data() -> ("Data"=w402:variant, "ModuleID"=w401:i32)  [unwired: 1 in]
        n158 = local read "Log Data"() -> (w403:bool)
        n159 = local read "btnPause"() -> (w404:bool)
        n160 = case shown="False" w404 {
          tunnel: w400 -> [w411 w431]
          tunnel: w399 -> [w410 w430]
          tunnel: [w409 w430] -> w397
          tunnel: [w408 w431] -> w398
          tunnel: w402 -> [w407 _]
          tunnel: w401 -> [w406 _]
          tunnel: w403 -> [w405 _]
          frame False {
            n161 = case shown="True" w405 {
              tunnel: w411 -> [w413 w421]
              tunnel: w410 -> [w412 w420]
              tunnel: [w412 w419] -> w409
              tunnel: [w413 w418] -> w408
              tunnel: w407 -> [_ w417]
              tunnel: w406 -> [_ w415]
              frame False {
              }
              frame True {
                n162 = local read "ModuleID"() -> (w414:i32)
                n163 = Equal?(x=w415, y=w414) -> (x = y?=w416:bool)
                n164 = case shown="True" w416 {
                  tunnel: [w422 w428] -> w419
                  tunnel: w421 -> [w423 w427]
                  tunnel: w420 -> [w422 w429]
                  tunnel: [w423 w425] -> w418
                  tunnel: w417 -> [_ w426]
                  frame False {
                  }
                  frame True {
                    n165 = call "VisEnqueueElement.vi"("Error Array In"=w429, "Data"=w426, "Message"="Log Parameter Set", "queue in"=w427) -> ("Error Array Out"=w428:errorcluster[], "queue out"=w425:refnum<queue>)  [unwired: 6 in]
                  }
                }
              }
            }
          }
          frame True {
          }
        }
      }
      event User Event {
        n166 = event-data() -> ("ModuleID"=w433:i32)  [unwired: 1 in, 5 out]
        n167 = local read "ModuleID"() -> (w432:i32)
        n168 = Equal?(x=w432, y=w433) -> (x = y?=w438:bool)
        n169 = case shown="True" w438 {
          tunnel: [w439 w444] -> w435
          tunnel: [w440 w443] -> w436
          tunnel: w437 -> [w440 w442]
          tunnel: w434 -> [w439 w441]
          frame False {
          }
          frame True {
            n170 = call "VisEnqueueElement.vi"("Priority? (F)"=TRUE, "Error Array In"=w441, "Message"="Stop", "queue in"=w442) -> ("Error Array Out"=w444:errorcluster[], "queue out"=w443:refnum<queue>)  [unwired: 6 in]
          }
        }
      }
      event "Display": Value Change {
        n171 = event-data() -> ("NewVal"=w450:enum16{"Raw Data", "Voltage Vs Current"})  [unwired: 1 in]
        n172 = case shown="\"Raw Data\", Default" w450 {
          tunnel: [TRUE FALSE] -> w449
          frame "Raw Data", Default {
          }
          frame "Voltage Vs Current" {
          }
        }
        n173 = Not(x=w449) -> (.not. x?=w448:bool)
        n174 = property on="Chart" class="WFChart (strict)"("Visible"=w449) -> ()  [unwired: 2 in, 2 out]
        n175 = property on="XY Graph" class="XYGraph (strict)"("Visible"=w448) -> ()  [unwired: 2 in, 2 out]
      }
      event "Voltage", "Current": Value Change {
        n176 = event-data() -> ("CtlRef"=w458:refnum<vi>)  [unwired: 1 in]
        n177 = property class="Bool"(reference=w458) -> ("Label.Text"=w453:string)  [unwired: 1 in, 2 out]
        n178 = call "VisEnqueueElement.vi"("Data"=w453, "Message"="Set Parameter", "queue in"=w455) -> ("Error Array Out"=w457:errorcluster[], "queue out"=w456:refnum<queue>)  [unwired: 7 in]
      }
      event User Event {
        n179 = event-data() -> ("ModuleID"=w460:i32, "Data"=w459:variant)  [unwired: 1 in]
        n180 = local read "ModuleID"() -> (w461:i32)
        n181 = Equal?(x=w461, y=w460) -> (x = y?=w466:bool)
        n182 = case shown="True" w466 {
          tunnel: w462 -> [w467 w473]
          tunnel: w463 -> [w468 w472]
          tunnel: [w467 w471] -> w464
          tunnel: [w468 w470] -> w465
          tunnel: w459 -> [_ w469]
          frame False {
          }
          frame True {
            (unwired) TRUE ("Priority? (F)")
            n183 = call "VisEnqueueElement.vi"("Error Array In"=w472, "Data"=w469, "Message"="GotSettings", "queue in"=w473) -> ("Error Array Out"=w470:errorcluster[], "queue out"=w471:refnum<queue>)  [unwired: 6 in]
          }
        }
      }
      event "btnStopModule": Value Change {
        n184 = event-data() -> ()  [unwired: 1 in, 1 out]
        n185 = local read "ModuleID"() -> (w478:i32)
        n186 = call "StatusUpdateByModID.vi"("Status"="User requested module stop", "Accessors:Module ID"=w478) -> ("error out"=w479:errorcluster)  [unwired: 9 in]
        n187 = flat-sequence {
          tunnel: [w481] -> w476
          tunnel: w479 -> [_]
          frame #0 {
            n188 = local read "PluginName"() -> (w480:string)
            n189 = call "GetSetTestClass.vi"() -> ("Test.lvclass"=w482:refnum<class "Test.lvclass">)  [unwired: 11 in]
            n190 = call "StopModByName.vi"("Module Name"=w480, "Test.lvclass"=w482) -> ("ErrorArray Out"=w481:errorcluster[])  [unwired: 4 in, 5 out]
          }
        }
      }
      event User Event {
        # "Framework requested visualization stop"
        n191 = event-data() -> ("Data"=w483:variant)  [unwired: 1 in]
        n192 = local read "PluginName"() -> (w484:string)
        n193 = Variant To Data(type="" ("Message"), Variant=w483) -> (data=w494:string, error out=w492:errorcluster)  [unwired: 1 in]
        n194 = call <userlib>:"AddError.vi"("Severity"="Inform", "Priority"=u8 3, "ErrorArray In"=w485, "error in (no error)"=w492) -> ("ErrorArray Out"=w491:errorcluster[])  [unwired: 6 in, 1 out]
        n195 = Equal?(x=w484, y=w494) -> (x = y?=w493:bool)
        n196 = case shown="True" w493 {
          tunnel: w488 -> [w497 w501]
          tunnel: [w496 w500] -> w486
          tunnel: w491 -> [w496 w499]
          tunnel: [w497 w498] -> w487
          frame False {
          }
          frame True {
            n197 = call "VisEnqueueElement.vi"("Priority? (F)"=TRUE, "Error Array In"=w499, "Message"="Stop", "queue in"=w501) -> ("Error Array Out"=w500:errorcluster[], "queue out"=w498:refnum<queue>)  [unwired: 6 in]
          }
        }
      }
      event "Chart": Shortcut Menu Activation? {
        n198 = event-data() -> ("CtlRef"=w507:refnum<vi>, "MenuRef"=w506:refnum<k9>, "Coords"=w505:T21)  [unwired: 1 in]
        n199 = local read "MeasChannels"() -> (w504:string[])
        n200 = call "Handle Chart Menu Activation.vi"("Channel Names"=w504, "Coords"=w505, "MenuRef"=w506, "CtlRef"=w507) -> ("Channel Index"=→"Chart#":i32)  [unwired: 7 in]
        n201 = event-data() -> ()  [unwired: 2 in, 1 out]
      }
      event "Chart": Shortcut Menu Selection (User) {
        n202 = event-data() -> ("ItemTag"=w513:string)  [unwired: 1 in]
        n203 = Match Pattern(string=w513, regular expression="Meas_") -> (after substring=w515:string, offset past match=w514:i32)  [unwired: 1 in, 2 out]
        n204 = case shown="Default" w514 {
          tunnel: w512 -> [w521 w524]
          tunnel: w511 -> [w520 w523]
          tunnel: [w519 w524] -> w510
          tunnel: [w518 w523] -> w509
          tunnel: w515 -> [w517 _]
          frame Default {
            # "User selected a measurement variable\nin the Chart shortcut menu"
            n205 = call "VisEnqueueElement.vi"("Error Array In"=w520, "Data"=w517, "Message"="Meas Variable Changed", "queue in"=w521) -> ("Error Array Out"=w518:errorcluster[], "queue out"=w519:refnum<queue>)  [unwired: 6 in]
          }
          frame -1 {
          }
        }
      }
    }
    n206 = call "VisEnqueueError.vi"("Error Array In"=w315, "Queue in"=w314) -> ("Error Array Out"=w316:errorcluster[], "Queue out"=w313:refnum<queue>)  [unwired: 8 in]
  }
  n207 = while {
    tunnel: w3 -> [w525]
    stop <- w526 stop-if-true
    # "Loop Parameters"
    n208 = event shown="[0] \"btnRunParamLoop\": Value Change" {
      selector: _ -> [_ _ _ _ _]
      dyn-events: _ -> [_ _ _ _ _]
      timeout: _ -> [_ _ _ _ _]
      tunnel: [_ _ _ _ TRUE] -> w526
      tunnel: w525 -> [_ _ _ _ _]
      event "btnRunParamLoop": Value Change {
        # "AcPwrLoopParameter,DC,Voltage,-1,7.5,0.25,2,5,#"
        # "Send parameter looping script"
        n209 = event-data() -> ()  [unwired: 1 in, 1 out]
        n210 = local read "Loop Parameters"() -> (w529:T1)
        n211 = local read "PluginName"() -> (w528:string)
        n212 = Unbundle By Name(w529) -> ("Parameter"=w540:T22, "Start Value"=w539:dbl, "Increment"=w538:dbl, "Interval (s)"=w537:dbl, "# Iterations"=w536:u32)
        n213 = Match Pattern(string=w528, regular expression="[.]") -> (after substring=w531:string)  [unwired: 1 in, 3 out]
        n214 = Format Into String(format string="AcPwrLoopParameter,%s,%s,-1,%#4g,%#4g,%#4g,%d,#%s", enum16{"AC", "DC"}."DC" ("input 1"), w540, w539, w538, w537, w536, w531) -> (resulting string=w527:string)  [unwired: 2 in, 1 out]
        n215 = invoke class="App" method="Clipboard.Write"("Param 0"=w527) -> ()  [unwired: 3 in, 4 out]
        n216 = Build Array(w527, "Stop" ("element")) -> (w533:string[])
        n217 = call "GetSetTestClass.vi"() -> ("Test.lvclass"=w532:refnum<class "Test.lvclass">)  [unwired: 11 in]
        n218 = call "ScriptedStateMachine.vi"("script"=w533, "Test.lvclass 2"=w532) -> ()  [unwired: 7 in, 3 out]
      }
      event "btnStopParameterLoop": Value Change {
        n219 = event-data() -> ()  [unwired: 1 in, 6 out]
      }
      event Value Change {
        n220 = event-data() -> ()  [unwired: 1 in, 1 out]
        n221 = Unbundle By Name("Loop Parameters") -> ("End Value"=w549:dbl, "Start Value"=w548:dbl, "# Iterations"=w546:u32)
        n222 = Decrement(x=w546) -> (x-1=w543:u32)
        n223 = Subtract(x=w549, y=w548) -> (x-y=w547:dbl)
        n224 = Divide(x=w547, y=w543) -> (x/y=w545:dbl)
        n225 = Bundle By Name(cluster="Loop Parameters", "Increment"=w545) -> (w544:T1)
        n226 = local write "Loop Parameters"(w544) -> ()
      }
      event Value Change {
        n227 = event-data() -> ()  [unwired: 1 in, 1 out]
        n228 = local read "Loop Parameters"() -> (w555:T1)
        n229 = Unbundle By Name(w555) -> ("End Value"=w558:dbl, "Start Value"=w557:dbl, "Increment"=w552:dbl)
        n230 = Subtract(x=w558, y=w557) -> (x-y=w556:dbl)
        n231 = Divide(x=w556, y=w552) -> (x/y=w554:dbl)
        n232 = Round Toward -Infinity(1:w554) -> (0:w551:dbl)
        n233 = Increment(x=w551) -> (x+1=w550:dbl)
        n234 = Bundle By Name(cluster=w555, "# Iterations"=w550) -> (w553:T1)
        n235 = local write "Loop Parameters"(w553) -> ()
      }
      event "ExitHelperLoops?": Value Change {
        n236 = event-data() -> ()  [unwired: 1 in, 1 out]
      }
    }
  }
  n237 = Unregister For Events(event registration refnum=w38) -> (error out=w36:errorcluster)  [unwired: 1 in]
  n238 = flat-sequence {
    tunnel: w10 -> [w561]
    tunnel: w9 -> [_]
    frame #0 {
      n239 = TDMS Close(11:w561) -> ()  [unwired: 1 in, 2 out]
      n240 = property on="ExitHelperLoops?" class="Bool (strict)"("Val(Sgnl)"=TRUE ("Value (Signaling)")) -> ()  [unwired: 2 in, 2 out]
    }
  }
  n241 = flat-sequence {
    tunnel: w36 -> [w565]
    tunnel: [w564] -> w34
    tunnel: w21 -> [w563]
    tunnel: w9 -> [_]
    frame #0 {
      n242 = Release Queue(queue=w563, force destroy? (F)=TRUE, error in (no error)=w565) -> (error out=w564:errorcluster)  [unwired: 2 out]
    }
  }
  n243 = Build Array (concatenate)(w37, w9) -> (w35:errorcluster[])
  n244 = call <userlib>:"AddError.vi"("ErrorArray In"=w35, "error in (no error)"=w34) -> ("ErrorArray Out"=w33:errorcluster[])  [unwired: 8 in, 1 out]
  n245 = disable-structure shown="Disabled" {
    disable-tunnel: w33 -> [w568 w574]
    disable-tunnel: w32 -> [w567 _]
    disable-tunnel: [w566 w574] -> w6
    frame Disabled {
      n246 = Cluster To Array(cluster=w567) -> (array=w569:refnum<user-event>[])
      n247 = for {
        tunnel: w569 -> [w573] mode=indexing
        shift-right: [w572] -> w566
        shift-left: w568 -> [w571]
        n248 = Destroy User Event(user event=w573) -> (error out=w570:errorcluster)  [unwired: 1 in]
        n249 = call <userlib>:"AddError.vi"("ErrorArray In"=w571, "error in (no error)"=w570) -> ("ErrorArray Out"=w572:errorcluster[])  [unwired: 8 in, 1 out]
      }
    }
    frame Enabled {
    }
  }
  "ErrorArray" <- w6
  n250 = Empty Array?(array=w6) -> (empty?=w31:bool)
  n251 = flat-sequence {
    tunnel: "PluginName" -> [w576]
    tunnel: w6 -> [_]
    frame #0 {
      n252 = call "VisDidStop.vi"("DidStop?"=TRUE, "Module Name"=w576) -> ()  [unwired: 9 in, 1 out]
    }
  }
  n253 = case shown="True" w31 {
    tunnel: [w577 _] -> w20
    tunnel: w6 -> [w578 _]
    frame False {
      n254 = Merge Errors(w578) -> (w577:errorcluster)
    }
    frame True {
      n255 = invoke class="VI" method="FP.Close"() -> ()  [unwired: 3 in, 3 out]
    }
  }
  n256 = call <vilib>:"Simple Error Handler.vi"("error in (no error)"=w20) -> ()  [unwired: 4 in, 5 out]
